vi "Set DAC Output.vi"(8 "error in (no error)":errorcluster, 9 "iValue":i32, 10 "iResolution":i32, 11 "iOption":i32) -> (0 "error out":errorcluster, 3 "function return":u32)   [LabVIEW 2014, in "atmcd32d.lvlib"]
doc: "unsigned int WINAPI SetDACOutput(int iOption, int iResolution, int iValue);"
uses:
  atmcd32d.lvlib
  atmcd32d.dll
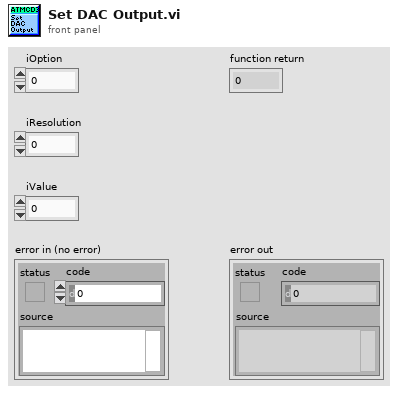
[diagram p1: front panel]
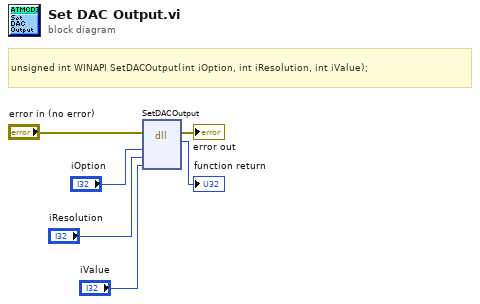
[diagram p0: block diagram]
diagram:
  # "unsigned int WINAPI SetDACOutput(int iOption, int iResolution, int iValue);"
  n1 = dll-call lib="C:/Users/Bakir/Documents/Lambda2-Testing/lib/Andorlib/atmcd32d.*" fn="SetDACOutput"(error in="error in (no error)", "iOption"="iOption", "iResolution"="iResolution", "iValue"="iValue") -> (error out=→"error out":errorcluster, →"function return":u32)  [unwired: 5 in, 1 out]
